vi "Code Alphabet.vi"() -> (2 "Code Alphabet":string="~-_.0123456789abcdefghijklmnopqrstuvwxyzABCDEFGHIJKLMNOPQRSTUVWXYZ")   [LabVIEW 2020, in "OAuth2.lvlib"]
doc: "Defines the default characters that can be used to randomly generate a Code Verifier string."
uses:
  OAuth2.lvlib
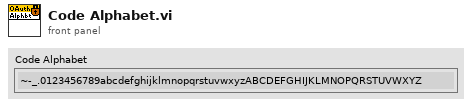
[diagram p1: front panel]
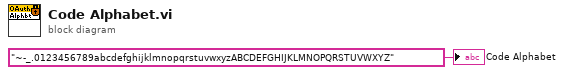
[diagram p0: block diagram]
diagram:
  "Code Alphabet" <- "~-_.0123456789abcdefghijklmnopqrstuvwxyzABCDEFGHIJKLMNOPQRSTUVWXYZ" ("Alphabet (Default)")
